vi "p2.vi"() -> ()   [LabVIEW 2023, in "d14.lvlib"]
uses:
  d14.lvlib
  AOC/AOC.lvlib
panel:
  out "Answer":i32
  in  "Example":string="O....#....\nO.OO#....#\n.....##...\nOO.#O....O\n.O.....O#.\nO.#..O.#.#\n..O..#O..O\n.......O..\n#....###..\n#OO..#...."
  in  "Example":bool
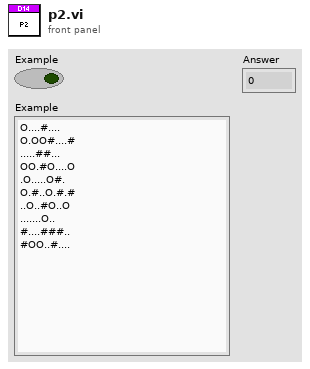
[diagram p1: front panel]
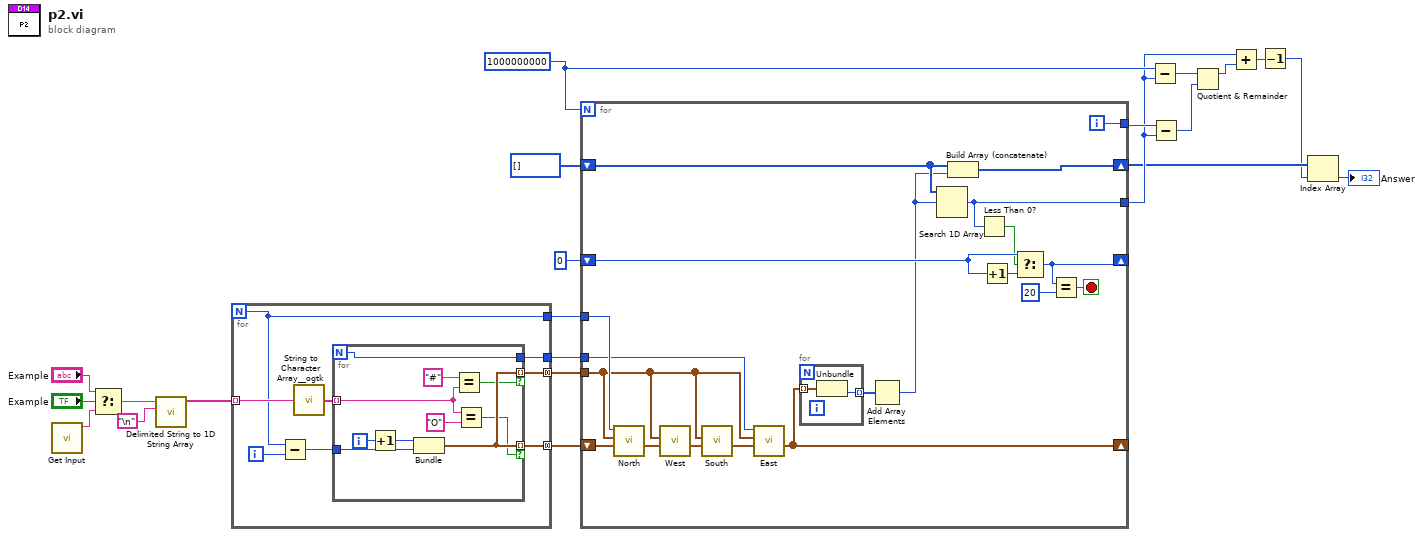
[diagram p0: block diagram]
diagram:
  w9 = 1000000000
  n1 = call "Get Input.vi"() -> ("Input"=w22:string)  [unwired: 11 in]
  n2 = Select(t="Example", s="Example", f=w22) -> (s? t:f=w19:string)
  n3 = call <vilib>:"Delimited String to 1D String Array.vi"("delimiter"="\n", "delimited string"=w19) -> ("string array"=w17:string[])  [unwired: 9 in]
  n4 = for {
    N -> [w25]
    tunnel: w17 -> [w30] mode=indexing
    tunnel: [w28] -> w13 mode=concatenating
    tunnel: [w27] -> w16 mode=concatenating
    tunnel: [w25] -> w15
    tunnel: [w23] -> w14
    i -> [w24]
    n5 = Subtract(x=w25, y=w24) -> (x-y=w26:i32)
    n6 = call <userlib>:"String to Character Array__ogtk.vi"("Input String"=w30) -> ("Character Array"=w29:string[])
    n7 = for {
      N -> [w31]
      tunnel: w29 -> [w35] mode=indexing
      tunnel: w26 -> [w39]
      tunnel: [w38] -> w27 mode=indexing if=w33
      tunnel: [w38] -> w28 mode=indexing if=w36
      tunnel: [w31] -> w23
      i -> [w40]
      n8 = Increment(x=w40) -> (x+1=w32:i32)
      n9 = Bundle(w32, w39) -> (w38:cluster{i32, i32})  [unwired: 1 in]
      n10 = Equal?(x="#", y=w35) -> (x = y?=w36:bool)
      n11 = Equal?(x=w35, y="O") -> (x = y?=w33:bool)
    }
  }
  n12 = for {
    N: w9 -> [_]
    tunnel: w15 -> [w59]
    tunnel: w14 -> [w58]
    tunnel: w13 -> [w54]
    shift-right: [w46] -> _
    shift-left: w16 -> [w60]
    shift-right: [w51] -> _
    shift-left: 0 -> [w53]
    shift-right: [w43] -> w3
    shift-left: i32[] [] -> [w45]
    tunnel: [w44] -> w5
    tunnel: [w41] -> w10
    i -> [w41]
    stop <- w49 stop-if-true
    n13 = call "North.vi"("Spheres in"=w60, "Cubes"=w54, "Northmost"=w59) -> ("Spheres out"=w57:cluster{i32, i32}[])  [unwired: 8 in]
    n14 = call "West.vi"("Spheres in"=w57, "Cubes"=w54) -> ("Spheres out"=w56:cluster{i32, i32}[])  [unwired: 9 in]
    n15 = call "South.vi"("Spheres in"=w56, "Cubes"=w54) -> ("Spheres out"=w55:cluster{i32, i32}[])  [unwired: 9 in]
    n16 = call "East.vi"("Spheres in"=w55, "Cubes"=w54, "Eastmost"=w58) -> ("Spheres out"=w46:cluster{i32, i32}[])  [unwired: 8 in]
    n17 = for {
      tunnel: w46 -> [w62] mode=indexing
      tunnel: [w61] -> w47 mode=indexing
      n18 = Unbundle(w62) -> (w61:i32)  [unwired: 1 out]
    }
    n19 = Add Array Elements(numeric array=w47) -> (sum=w42:i32)
    n20 = Search 1D Array(1D array=w45, element=w42) -> (index of element=w44:i32)  [unwired: 1 in]
    n21 = Build Array (concatenate)(w45, w42) -> (w43:i32[])
    n22 = Less Than 0?(x=w44) -> (x < 0?=w48:bool)
    n23 = Increment(x=w53) -> (x+1=w52:i32)
    n24 = Select(t=w53, s=w48, f=w52) -> (s? t:f=w51:i32)
    n25 = Equal?(x=w51, y=20) -> (x = y?=w49:bool)
  }
  n26 = Subtract(x=w9, y=w5) -> (x-y=w8:i32)
  n27 = Subtract(x=w10, y=w5) -> (x-y=w7:i32)
  n28 = Quotient & Remainder(x=w8, y=w7) -> (x-y*floor(x/y)=w6:i32)  [unwired: 1 out]
  n29 = Add(x=w5, y=w6) -> (x+y=w4:i32)
  n30 = Decrement(x=w4) -> (x-1=w2:i32)
  n31 = Index Array(array=w3, index=w2) -> (element=→"Answer":i32)
